vi "RunNumberGlobal.vi"() -> ()   [LabVIEW 2018]
panel:
  in  "RunNumber":dbl
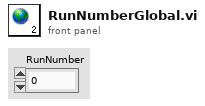
[diagram p1: front panel]
diagram:
